vi "GLIMPSE Fetch Image.vi"(4 "Display FOV number":i16(slide) scale=0.0..10.0, 5 "Total FOVs":i16, 6 "Header file data":T1 {"Pixel depth" items=["8 bits", "16 bits", "Float", "Complex", "RGB", "HSL"]; "time of 1st frame, \nsec since 1/1/04" format="%.2f"}, 7 "Acqisition files refnums":refnum<file>[](array[refnum]), 8 "error in":errorcluster, 10 "Logical Frame Number\n(starting with zero)":u32, 11 "Image In":T5) -> (0 "error out":errorcluster, 3 "Image Out":T5)   [LabVIEW 2016]
doc: "Returns the time value and image data for a particular stored image (field or frame) in a sequence. For use outside of Glimpse, the vi should be replaced with the user's routine to fetch the data."
uses:
  <vilib>/vision/Image Controls.llb/IMAQ Image.ctl
  Header file data.ctl
  Seq file v 1/Offset table.ctl
  Seq file v 1/Offset.ctl
  Seq file v 1/file number.ctl
  GLIMPSE Globals.vi
  <vilib>/vision/NI_Vision_Development_Module.lvlib
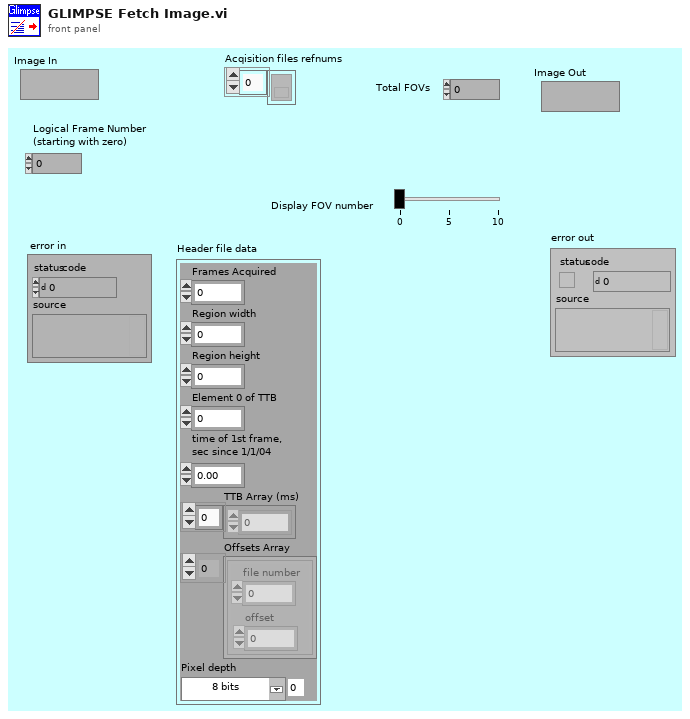
[diagram p1: front panel]
types:
  T1 = typedef "Header file data.ctl" = cluster{"Frames Acquired":u32, "Region width":i32, "Region height":i32, "Element 0 of TTB":u32, "time of 1st frame, \nsec since 1/1/04":dbl, "TTB Array (ms)":u32[], "Offsets Array":T2, "Pixel depth":u32}
  T2 = typedef "Offset table.ctl" = cluster{"offset":T3, "file number":T4}[]
  T3 = typedef "Offset.ctl" = i32
  T4 = typedef "file number.ctl" = u8
  T5 = typedef "IMAQ Image.ctl" = refnum<image>
  T6 = enum16{"Frames", "Fields, Odd 1st", "Fields, Even 1st", "Fields, Averaged"}
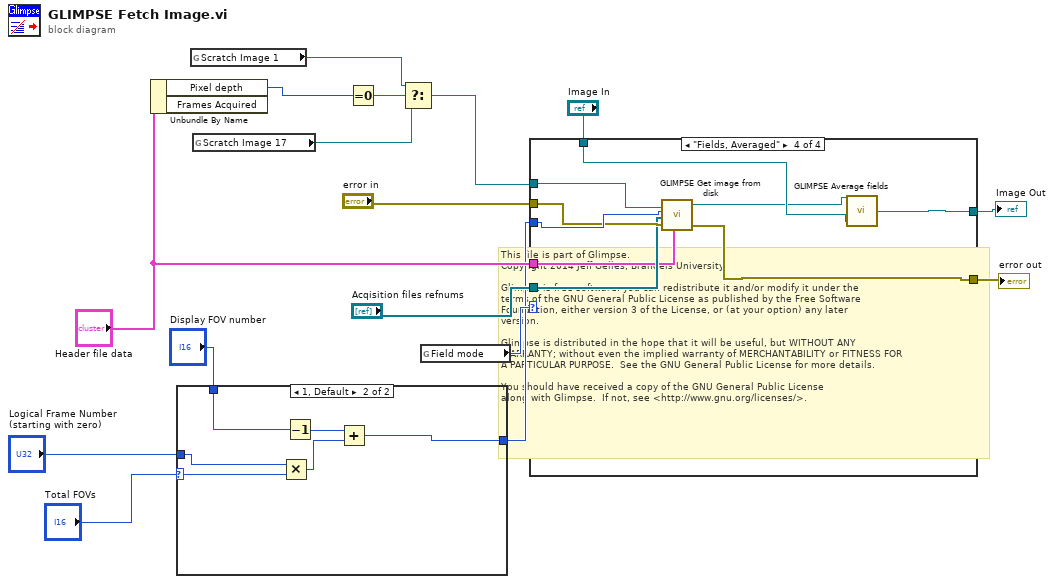
[diagram p0: block diagram]
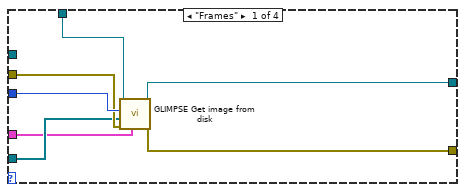
[diagram p3: hidden frame]
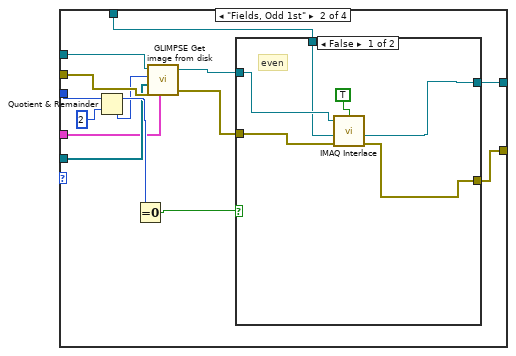
[diagram p4: hidden frame]
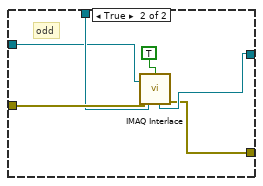
[diagram p5: hidden frame]
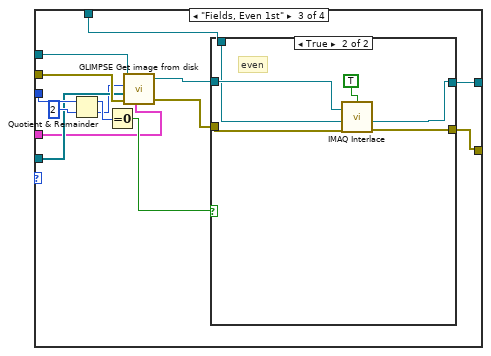
[diagram p6: hidden frame]
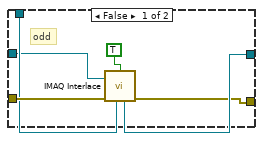
[diagram p7: hidden frame]
diagram:
  # "This file is part of Glimpse. \nCopyright 2014 Jeff Gelles, Brandeis University.    \n\nGlimpse is free software: you can redistribute it and/or modify it under the \nterms of the GNU General Public License as published by the Free Software \nFoundation, either version 3 of the License, or (at your option) any later \nversion.\n\nGlimpse is distributed in the hope that it will be useful, but WITHOUT ANY \nWARRANTY; without even the implied warranty of MERCHANTABILITY or FITNESS FOR \nA PARTICULAR PURPOSE.  See the GNU General Public License for more details.\n\nYou should have received a copy of the GNU General Public License\nalong with Glimpse.  If not, see <http://www.gnu.org/licenses/>."
  n1 = Unbundle By Name("Header file data") -> ("Pixel depth"=w6:u32)  [unwired: 1 out]
  n2 = case shown="1, Default" "Total FOVs" {
    selector: "Total FOVs" -> [_ w22]
    tunnel: "Logical Frame Number\n(starting with zero)" -> [w17 w23]
    tunnel: [w17 w20] -> w2
    tunnel: "Display FOV number" -> [_ w18]
    frame 0 {
    }
    frame 1, Default {
      n3 = Multiply(x=w23, y=w22) -> (x*y=w21:u32)
      n4 = Decrement(x=w18) -> (x-1=w19:i16)
      n5 = Add(x=w19, y=w21) -> (x+y=w20:u32)
    }
  }
  n6 = global read "GLIMPSE Globals.vi" "Scratch Image 1"() -> (w9:T5)
  n7 = global read "GLIMPSE Globals.vi" "Scratch Image 17"() -> (w8:T5)
  n8 = Equal To 0?(x=w6) -> (x = 0?=w10:bool)
  n9 = Select(t=w9, s=w10, f=w8) -> (s? t:f=w7:T5)
  n10 = global read "GLIMPSE Globals.vi" "Field mode"() -> (w14:T6)
  n11 = case shown="\"Fields, Averaged\"" w14 {
    tunnel: [w27 w41 w66 w91] -> w16
    tunnel: w2 -> [w30 w44 w70 w90]
    tunnel: "Image In" -> [w28 w35 w62 w87]
    tunnel: "error in" -> [w29 w40 w65 w89]
    tunnel: [w26 w39 w63 w88] -> w12
    tunnel: "Acqisition files refnums" -> [w25 w34 w60 w85]
    tunnel: w7 -> [_ w32 w58 w84]
    tunnel: "Header file data" -> [w24 w31 w57 w83]
    frame "Frames" {
      n12 = call "GLIMPSE Get image from disk.vi"("Header file data"=w24, "error in"=w29, "Acqisition files refnums"=w25, "Physical Frame Number\n(Starting with zero)"=w30, "Image buffer in"=w28) -> ("error out"=w26:errorcluster, "Image out"=w27:T5)  [unwired: 4 out]
    }
    frame "Fields, Odd 1st" {
      n13 = Quotient & Remainder(x=w44, y=u32 2) -> (x-y*floor(x/y)=w38:u32, floor(x/y)=w33:u32)
      n14 = Equal To 0?(x=w38) -> (x = 0?=w42:bool)
      n15 = call "GLIMPSE Get image from disk.vi"("Header file data"=w31, "error in"=w40, "Acqisition files refnums"=w34, "Physical Frame Number\n(Starting with zero)"=w33, "Image buffer in"=w32) -> ("error out"=w37:errorcluster, "Image out"=w36:T5)  [unwired: 4 out]
      n16 = case shown="False" w42 {
        tunnel: [w50 w56] -> w41
        tunnel: w37 -> [w47 w55]
        tunnel: [w49 w54] -> w39
        tunnel: w36 -> [w46 w51]
        tunnel: w35 -> [w45 w52]
        frame False {
          # "even"
          n17 = call "IMAQ Interlace"("error in (no error)"=w47, "Image Even"=w45, "Image Frame"=w46, "Interlace/Separate (Interlace)"=TRUE) -> ("Image Even Out"=w50:T5, "error out"=w49:errorcluster)  [unwired: 1 in, 2 out]
        }
        frame True {
          # "odd"
          n18 = call "IMAQ Interlace"("error in (no error)"=w55, "Image Odd"=w52, "Image Frame"=w51, "Interlace/Separate (Interlace)"=TRUE) -> ("Image Odd Out"=w56:T5, "error out"=w54:errorcluster)  [unwired: 1 in, 2 out]
        }
      }
    }
    frame "Fields, Even 1st" {
      n19 = Quotient & Remainder(x=w70, y=2) -> (x-y*floor(x/y)=w68:u32, floor(x/y)=w59:u32)
      n20 = Equal To 0?(x=w68) -> (x = 0?=w67:bool)
      n21 = call "GLIMPSE Get image from disk.vi"("Header file data"=w57, "error in"=w65, "Acqisition files refnums"=w60, "Physical Frame Number\n(Starting with zero)"=w59, "Image buffer in"=w58) -> ("error out"=w64:errorcluster, "Image out"=w61:T5)  [unwired: 4 out]
      n22 = case shown="True" w67 {
        tunnel: [w76 w82] -> w66
        tunnel: w62 -> [w72 w77]
        tunnel: w64 -> [w73 w80]
        tunnel: [w74 w79] -> w63
        tunnel: w61 -> [w71 w78]
        frame False {
          # "odd"
          n23 = call "IMAQ Interlace"("error in (no error)"=w73, "Image Odd"=w72, "Image Frame"=w71, "Interlace/Separate (Interlace)"=TRUE) -> ("Image Odd Out"=w76:T5, "error out"=w74:errorcluster)  [unwired: 1 in, 2 out]
        }
        frame True {
          # "even"
          n24 = call "IMAQ Interlace"("error in (no error)"=w80, "Image Even"=w77, "Image Frame"=w78, "Interlace/Separate (Interlace)"=TRUE) -> ("Image Even Out"=w82:T5, "error out"=w79:errorcluster)  [unwired: 1 in, 2 out]
        }
      }
    }
    frame "Fields, Averaged" {
      n25 = call "GLIMPSE Get image from disk.vi"("Header file data"=w83, "error in"=w89, "Acqisition files refnums"=w85, "Physical Frame Number\n(Starting with zero)"=w90, "Image buffer in"=w84) -> ("error out"=w88:errorcluster, "Image out"=w86:T5)  [unwired: 4 out]
      n26 = call "GLIMPSE Average fields.vi"("Field buffer In"=w87, "Image in"=w86) -> ("Field buffer Out"=w91:T5)
    }
  }
  "Image Out" <- w16
  "error out" <- w12
